vi "Plugin_SpecPage.vi"(10 "Spec Page Interface":T6, 11 "MetaDataObj in":refnum<class "MetaDataObj.lvclass">) -> (3 "MetaDataObj out":refnum<class "MetaDataObj.lvclass">)   [LabVIEW 2021, in "CIF_Plugin_Generator.lvclass"]
uses:
  CIF_Plugin_Generator.lvclass
  <vilib>/CIF Foundation/CIF LabVIEW Scripting/LV Scripting/LV Scripting Utilities.lvlib
  C:/Program Files/National Instruments/LabVIEW 2021/resource/dialog/NewProjectWizard/MetaDataObj/MetaDataObj.lvclass
  C:/Program Files/National Instruments/LabVIEW 2021/ProjectTemplates/Source/CIF/Plugin Generator/CIF_Plugin_Generator.lvclass
  <resource>/dialog/NewProjectWizard/Spec Page Interface.ctl
  <resource>/dialog/NewProjectWizard/MetaDataObj/MetaDataObj.lvclass
  <vilib>/CIF Foundation/CIF LabVIEW Scripting/LV Scripting/Typedef/Icon Overlay.ctl
  <vilib>/CIF Foundation/CIF Channels Core/CIFChannels/Typedef/Direction.ctl
  <vilib>/CIF Foundation/CIF Channels Core/CIFChannels/CIFChannels.lvclass
  <vilib>/CIF Foundation/CIF Core/Channels/ChannelRegistrar/typedef/Registered Channel Types.ctl
  <vilib>/CIF Foundation/CIF Core/Channels/ChannelRegistrar/ChannelRegistrar.lvlib
  <vilib>/CIF Foundation/CIF Core/Channels/ChannelRegistrar/typedef/Channel Definition for Scripting.ctl
  Typedef/Documentation Info.ctl
  Plugin Generator.lvlib
panel:
  in  "Documentation":T1
  in  "Channels to Create":T2[](array[typedef])
  in  "Plugin Name":string
  in  "Root Directory":path
  out "Icon":picture
  in  "Icon Customization":T5={"Text"="Plugin", "Background color"=7208704, "Text color"=0}
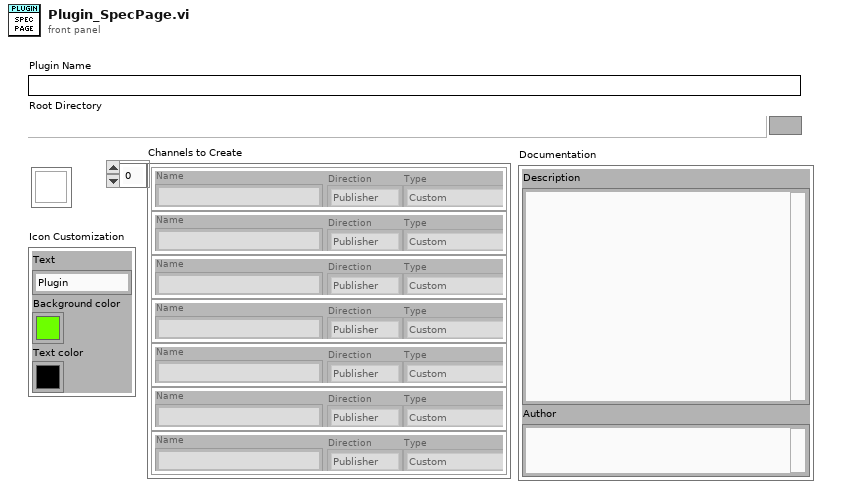
[diagram p1: front panel]
types:
  T1 = typedef "Plugin Generator.lvlib/Documentation Info.ctl" = cluster{"Description":string, "Author":string}
  T2 = typedef "ChannelRegistrar.lvlib/Channel Definition for Scripting.ctl" = cluster{"Name":string, "Direction":T3, "Type":T4}
  T3 = typedef "CIFChannels.lvclass/Direction.ctl" = enum16{"Publisher", "Subscriber"}
  T4 = typedef "ChannelRegistrar.lvlib/Registered Channel Types.ctl" = enum16{"Custom", "Double_Tag", "I64_Tag", "U64_Tag", "U8_FIFO", "CAN_FIFO", "L2Enet_FIFO", "DAQ_FIFO", "Universal_FIFO", "String_Tag"}
  T5 = typedef "LV Scripting Utilities.lvlib/Icon Overlay.ctl" = cluster{"Text":string, "Background color":u32, "Text color":u32}
  T6 = typedef "Spec Page Interface.ctl" = cluster{"\"Tab Forward To\" Refnum":refnum<vi>, "\"Tab Backward To\" Refnum":refnum<vi>, "Errors":refnum<user-event>, "Quit":refnum<user-event>}
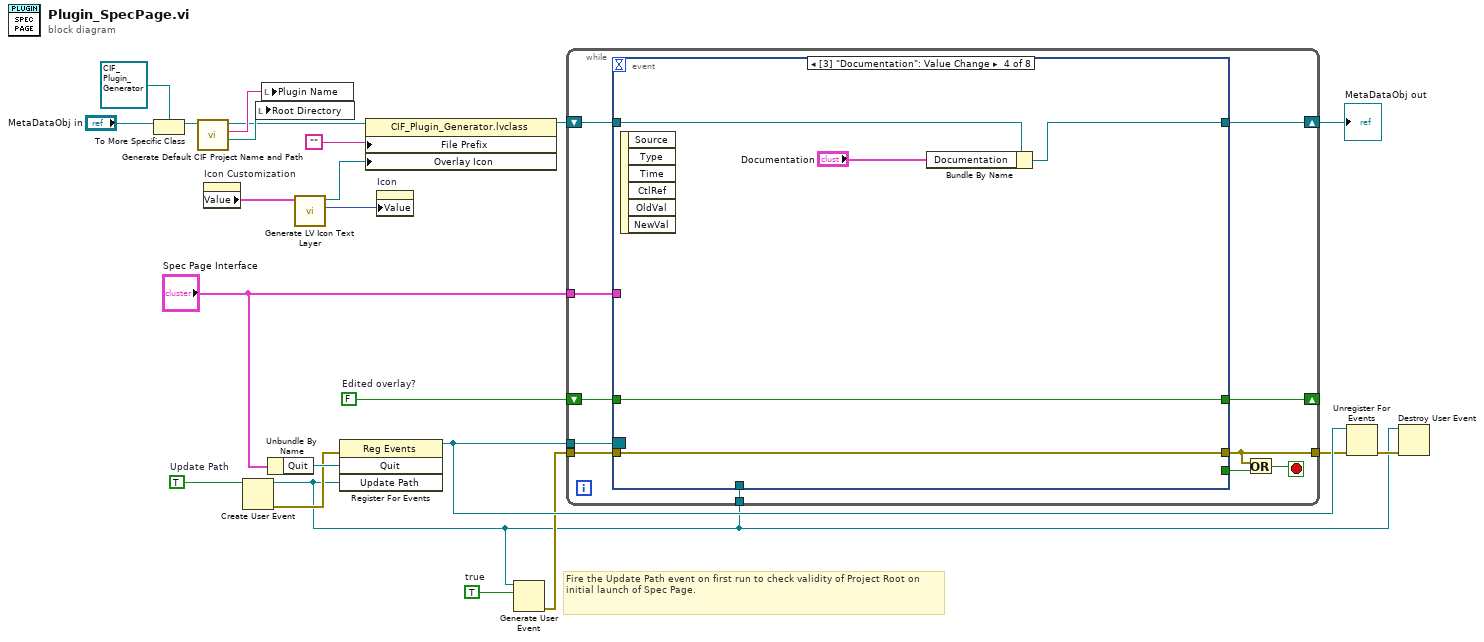
[diagram p0: block diagram]
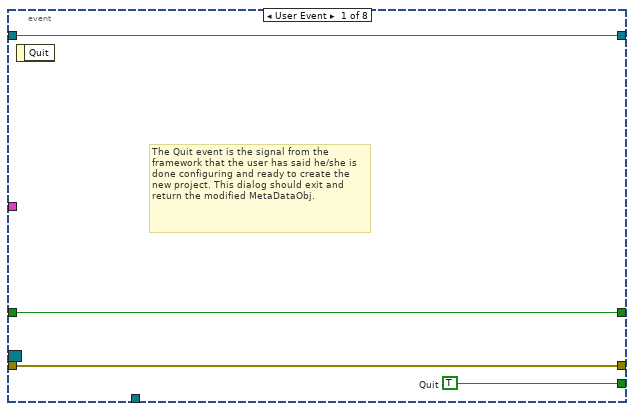
[diagram p2: hidden frame]
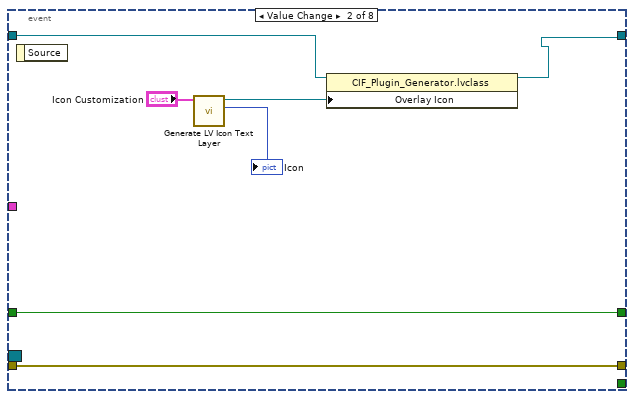
[diagram p3: hidden frame]
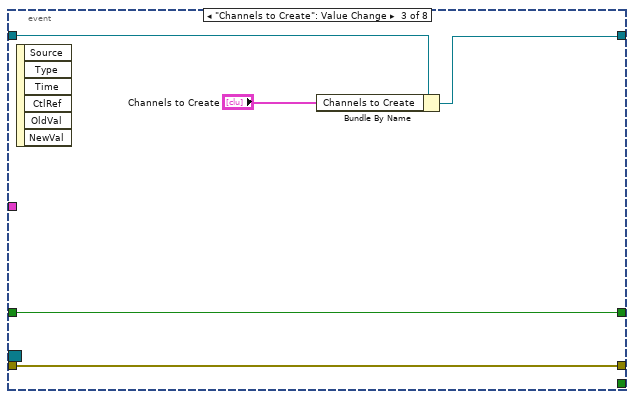
[diagram p4: hidden frame]
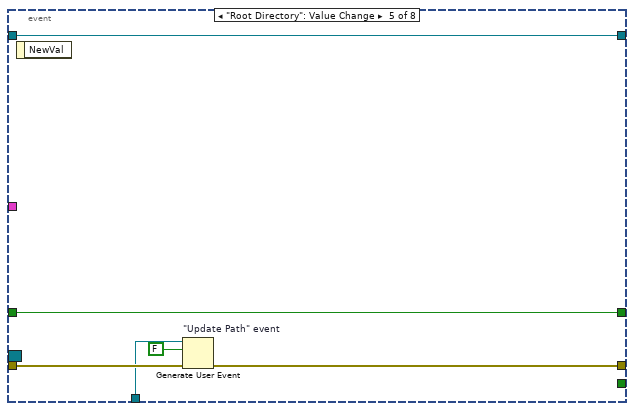
[diagram p5: hidden frame]
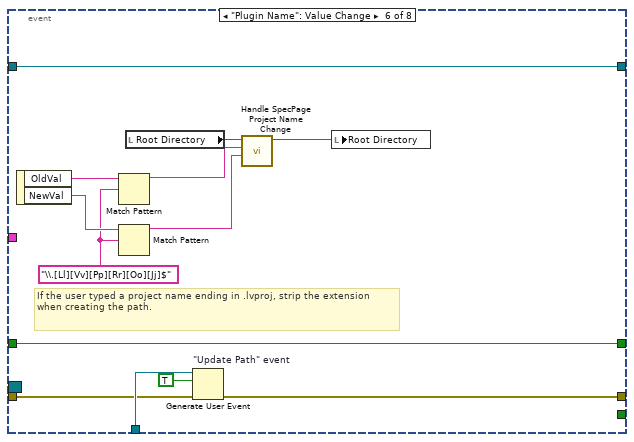
[diagram p6: hidden frame]
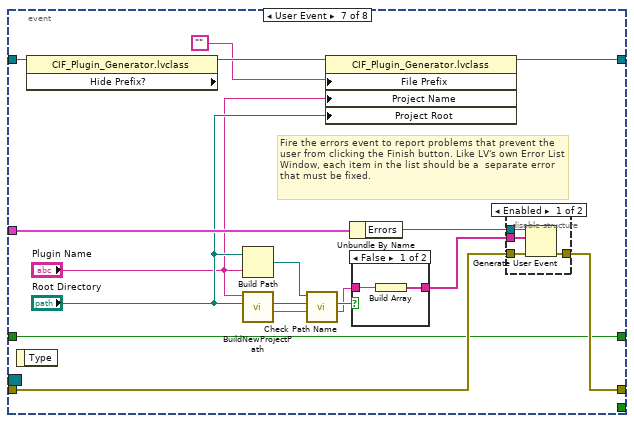
[diagram p7: hidden frame]
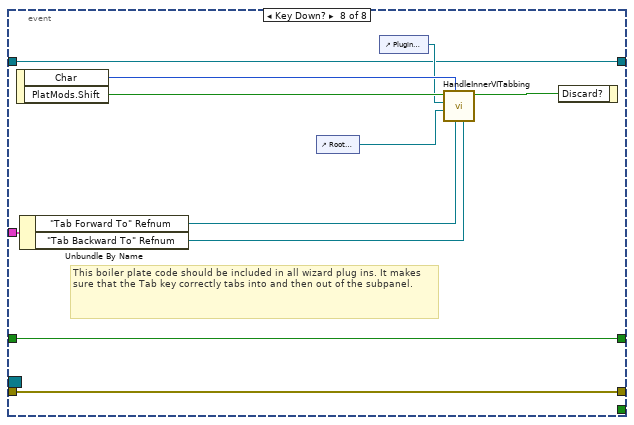
[diagram p10: hidden frame]
diagram:
  w6 = TRUE  # true
  w15 = FALSE  # Edited overlay?
  w19 = TRUE  # Update Path
  # "Fire the Update Path event on first run to check validity of Project Root on initial launch of Spec Page."
  n1 = To More Specific Class(target class=refnum<class "CIF_Plugin_Generator.lvclass"> refnum ("Plugin_Generator.lvclass"), reference="MetaDataObj in") -> (specific class reference=w2:refnum<class "CIF_Plugin_Generator.lvclass">)  [unwired: 1 in, 1 out]
  n2 = call "Generate Default CIF Project Name and Path.vi"("MetaDataObj in"=w2) -> ("Project Root"=w4:path, "Project Name"=w5:string, "MetaDataObj out"=w1:refnum<class "CIF_Plugin_Generator.lvclass">)  [unwired: 8 in]
  n3 = property on="Icon Customization" class="Clust (strict)"() -> ("Value"=w11:T5)  [unwired: 2 in, 2 out]
  n4 = Create User Event(user event datatype=w19) -> (user event=w13:refnum<user-event>, error out=w18:errorcluster)  [unwired: 1 in]
  n5 = local write "Root Directory"(w4) -> ()
  n6 = local write "Plugin Name"(w5) -> ()
  n7 = Unbundle By Name("Spec Page Interface") -> ("Quit"=w23:refnum<user-event>)
  n8 = call <vilib>:"Generate LV Icon Text Layer.vi"("Icon Overlay"=w11) -> ("Picture"=w10:picture, "Icon.lvlclass out"=w9:refnum<class "Icon.lvclass">)  [unwired: 8 in, 1 out]
  n9 = register-events(error in=w18, w23, w13) -> (reference out=w22:refnum<event-registration>)  [unwired: 1 in, 1 out]
  n10 = property class="CIF_Plugin_Generator.lvclass"(reference=w1, "File Prefix"="", "Overlay Icon"=w9) -> (reference out=w7:refnum<class "CIF_Plugin_Generator.lvclass">)  [unwired: 1 in, 1 out]
  n11 = property on="Icon" class="Pict"("Value"=w10) -> ()  [unwired: 2 in, 2 out]
  n12 = Generate User Event ("\"Update Path\" event")(user event=w13, event data cluster=w6) -> (error out=w14:errorcluster)  [unwired: 2 in, 1 out]
  n13 = while {
    tunnel: "Spec Page Interface" -> [w32]
    shift-right: [w31] -> w16
    shift-left: w7 -> [w30]
    tunnel: w22 -> [w34]
    tunnel: w14 -> [w33]
    tunnel: [w27] -> w20
    tunnel: w13 -> [w26]
    shift-right: [w24] -> _
    shift-left: w15 -> [w25]
    stop <- w29 stop-if-true
    n14 = event shown="[3] \"Documentation\": Value Change" {
      selector: w34 -> [_ _ _ _ _ _ _ _]
      dyn-events: _ -> [_ _ _ _ _ _ _ _]
      timeout: _ -> [_ _ _ _ _ _ _ _]
      tunnel: w32 -> [_ _ _ _ _ _ w89 w105]
      tunnel: [w38 _ _ _ _ _ _ _] -> w28
      tunnel: [w37 w45 w50 w55 w59 w70 w87 w102] -> w27
      tunnel: w33 -> [w37 w45 w50 w55 w60 w71 w88 w102]
      tunnel: [w36 w41 w47 w51 w61 w67 w85 w101] -> w31
      tunnel: w30 -> [w36 w42 w48 w53 w61 w67 w86 w101]
      tunnel: w26 -> [_ _ _ _ w58 w72 _ _]
      tunnel: w25 -> [w35 w44 w49 w54 w56 w68 w84 w100]
      tunnel: [w35 w44 w49 w54 w56 w68 w84 w100] -> w24
      event User Event {
        w38 = TRUE  # Quit
        # "The Quit event is the signal from the framework that the user has said he/she is done configuring and ready to create the new project. This dialog should exit and return the modified MetaDataObj."
        n15 = event-data() -> ()  [unwired: 1 in, 1 out]
      }
      event Value Change {
        n16 = event-data() -> ()  [unwired: 1 in, 1 out]
        n17 = call <vilib>:"Generate LV Icon Text Layer.vi"("Icon Overlay"="Icon Customization") -> ("Picture"=→"Icon":picture, "Icon.lvlclass out"=w43:refnum<class "Icon.lvclass">)  [unwired: 8 in, 1 out]
        n18 = property class="CIF_Plugin_Generator.lvclass"(reference=w42, "Overlay Icon"=w43) -> (reference out=w41:refnum<class "CIF_Plugin_Generator.lvclass">)  [unwired: 1 in, 1 out]
      }
      event "Channels to Create": Value Change {
        n19 = event-data() -> ()  [unwired: 1 in, 6 out]
        n20 = Bundle By Name(cluster=w48, "Channels to Create"="Channels to Create") -> (w47:refnum<class "CIF_Plugin_Generator.lvclass">)
      }
      event Value Change {
        n21 = event-data() -> ()  [unwired: 1 in, 6 out]
        n22 = Bundle By Name(cluster=w53, "Documentation"="Documentation") -> (w51:refnum<class "CIF_Plugin_Generator.lvclass">)
      }
      event "Root Directory": Value Change {
        n23 = event-data() -> ()  [unwired: 1 in, 1 out]
        n24 = Generate User Event "\"Update Path\" event"(user event=w58, event data cluster=FALSE ("event data"), error in=w60) -> (error out=w59:errorcluster)  [unwired: 1 in, 1 out]
      }
      event "Plugin Name": Value Change {
        w62 = "\\.[Ll][Vv][Pp][Rr][Oo][Jj]$" ("regular expression")
        # "If the user typed a project name ending in .lvproj, strip the extension when creating the path."
        n25 = event-data() -> ("OldVal"=w64:string, "NewVal"=w66:string)  [unwired: 1 in]
        n26 = Match Pattern(string=w64, regular expression=w62) -> (before substring=w63:string)  [unwired: 1 in, 3 out]
        n27 = Match Pattern(string=w66, regular expression=w62) -> (before substring=w65:string)  [unwired: 1 in, 3 out]
        n28 = local read "Root Directory"() -> (w74:path)
        n29 = Generate User Event "\"Update Path\" event"(user event=w72, event data cluster=TRUE ("event data"), error in=w71) -> (error out=w70:errorcluster)  [unwired: 1 in, 1 out]
        n30 = call <resource>:"Handle SpecPage Project Name Change.vi"("Project Name New Value"=w65, "Project Name Old Value"=w63, "Project Root in"=w74) -> ("Project Root out"=w73:path)  [unwired: 8 in]
        n31 = local write "Root Directory"(w73) -> ()
      }
      event User Event {
        # "Fire the errors event to report problems that prevent the user from clicking the Finish button. Like LV's own Error List Window, each item in the list should be a  separate error that must be fixed."
        n32 = event-data() -> ()  [unwired: 1 in, 1 out]
        n33 = property class="CIF_Plugin_Generator.lvclass" props=["Hide Prefix?"](reference=w86) -> (reference out=w83:refnum<class "CIF_Plugin_Generator.lvclass">)  [unwired: 1 in, 2 out]
        n34 = Build Path(base path="Root Directory", name or relative path="Plugin Name") -> (appended path=w75:path)
        n35 = call <resource>:"BuildNewProjectPath.vi"("Project Root"="Root Directory", "Project Name"="Plugin Name") -> ("Error Message"=w80:string, "Valid?"=w81:bool)  [unwired: 7 in, 1 out]
        n36 = call "Check Path Name.vi"("Error Message in"=w80, "Valid in"=w81, "New Project Path"=w75) -> ("Error Message out"=w78:string, "Valid out"=w79:bool)  [unwired: 7 in]
        n37 = property class="CIF_Plugin_Generator.lvclass"(reference=w83, "File Prefix"="", "Project Name"="Plugin Name", "Project Root"="Root Directory") -> (reference out=w85:refnum<class "CIF_Plugin_Generator.lvclass">)  [unwired: 1 in, 1 out]
        n38 = Unbundle By Name(w89) -> ("Errors"=w91:refnum<user-event>)
        n39 = case shown="False" w79 {
          tunnel: w78 -> [w98 _]
          tunnel: [w97 _] -> w90
          frame False {
            n40 = Build Array(w98) -> (w97:string[])
          }
          frame True {
          }
        }
        n41 = disable-structure shown="Enabled" {
          disable-tunnel: w91 -> [w95 _]
          disable-tunnel: w90 -> [w94 _]
          disable-tunnel: w88 -> [w93 w96]
          disable-tunnel: [w92 w96] -> w87
          frame Enabled {
            n42 = Generate User Event(user event=w95, event data cluster=w94, error in=w93) -> (error out=w92:errorcluster)  [unwired: 1 in, 1 out]
          }
          frame Disabled {
          }
        }
      }
      event Key Down? {
        # "This boiler plate code should be included in all wizard plug ins. It makes sure that the Tab key correctly tabs into and then out of the subpanel."
        n43 = event-data() -> ("Char"=w108:i16, "PlatMods.Shift"=w107:bool)  [unwired: 1 in]
        n44 = Unbundle By Name(w105) -> ("\"Tab Forward To\" Refnum"=w104:refnum<vi>, "\"Tab Backward To\" Refnum"=w103:refnum<vi>)
        n45 = control-ref of="Root Directory"() -> (w99:refnum<vi>)
        n46 = control-ref of="Plugin Name"() -> (w106:refnum<vi>)
        n47 = call <resource>:"HandleInnerVITabbing.vi"("Tab Backward To"=w103, "Tab Forward To"=w104, "Char"=w108, "Last Control"=w99, "First Control"=w106, "Shift"=w107) -> ("Discard"=w109:bool)  [unwired: 5 in]
        n48 = event-data("Discard?"=w109) -> ()  [unwired: 1 in, 1 out]
      }
    }
    n49 = Or(x=w27, y=w28) -> (x .or. y?=w29:bool)
  }
  "MetaDataObj out" <- w16
  n50 = Unregister For Events(event registration refnum=w22, error in=w20) -> (error out=w17:errorcluster)
  n51 = Destroy User Event(user event=w13, error in=w17) -> ()  [unwired: 1 out]
